vi "Resistance Change Benchmark.vi"() -> ()   [LabVIEW 2017]
uses:
  Source/NI 272x Resistive Simulation Custom Device Engine.lvlib
panel:
  out "Array 2":dbl[](array[numeric])
  out "Array":string[](array[string])
  out "average":dbl
  out "duration":u32
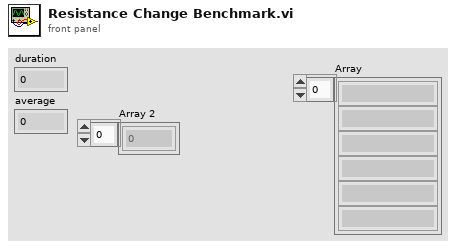
[diagram p1: front panel]
types:
  T1 = typedef "ni272x Reference.ctl" = refnum<k20>
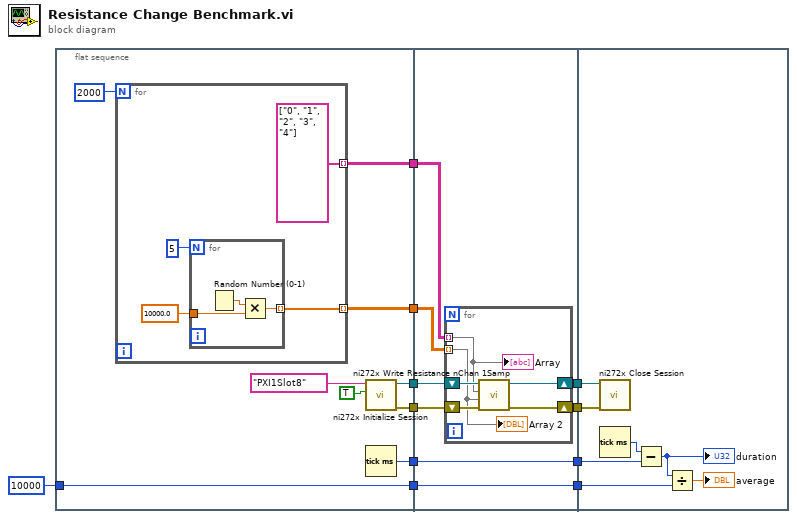
[diagram p0: block diagram]
diagram:
  n1 = flat-sequence {
    tunnel: [w20] -> w11
    tunnel: [w19] -> w10
    tunnel: 10000 -> [w16]
    tunnel: [w18] -> w7
    tunnel: [w17] -> w6
    tunnel: [w16] -> w4
    tunnel: [w12] -> w1
    tunnel: w11 -> [w33]
    tunnel: w10 -> [w31]
    tunnel: [w30] -> w9
    tunnel: w7 -> [w28]
    tunnel: w6 -> [w35]
    tunnel: [w35] -> w5
    tunnel: w4 -> [w34]
    tunnel: [w34] -> w3
    tunnel: [w32] -> w2
    tunnel: w1 -> [w29]
    tunnel: w9 -> [w47]
    tunnel: w5 -> [w45]
    tunnel: w3 -> [w43]
    tunnel: w2 -> [w48]
    frame #0 {
      n2 = for {
        N: 2000 -> [_]
        tunnel: [w23] -> w18 mode=indexing
        tunnel: [string[] ["0", "1", "2", "3", "4"]] -> w12 mode=indexing
        n3 = for {
          N: 5 -> [_]
          tunnel: 10000.0 ("y") -> [w26]
          tunnel: [w25] -> w23 mode=indexing
          n4 = Random Number (0-1)() -> (number: 0 to 1=w27:dbl)
          n5 = Multiply(x=w27, y=w26) -> (x*y=w25:dbl)
        }
      }
      n6 = call <instrlib>:"ni272x Initialize Session.vi"("reset device (T)"=TRUE, "DAQmx Device Name"=tag "PXI1Slot8") -> ("error out"=w19:errorcluster, "instrument handle out"=w20:T1)  [unwired: 8 in]
      n7 = Tick Count (ms)() -> (millisecond timer value=w17:u32)
    }
    frame #1 {
      n8 = for {
        shift-right: [w40] -> w32
        shift-left: w33 -> [w41]
        shift-right: [w38] -> w30
        shift-left: w31 -> [w39]
        tunnel: w29 -> [w37] mode=indexing
        tunnel: w28 -> [w36] mode=indexing
        n9 = call "ni272x Write Resistance nChan 1Samp.vi"("error in (no error)"=w39, "requested resistances (ohms)"=w36, "resistor channels"=w37, "instrument handle"=w41) -> ("error out"=w38:errorcluster, "instrument handle out"=w40:T1)  [unwired: 5 in, 1 out]
        "Array" <- w37
        "Array 2" <- w36
      }
    }
    frame #2 {
      n10 = call <instrlib>:"ni272x Close Session.vi"("error in (no error)"=w47, "instrument handle"=w48) -> ()  [unwired: 9 in, 1 out]
      n11 = Tick Count (ms)() -> (millisecond timer value=w46:u32)
      n12 = Subtract(x=w46, y=w45) -> (x-y=w44:u32)
      "duration" <- w44
      n13 = Divide(x=w44, y=w43) -> (x/y=→"average":dbl)
    }
  }
